vi "Query Current.vi"(8 "error in (no error)":errorcluster, 11 "Manual PSU in":refnum<class "Manual PSU.lvclass">) -> (0 "error out":errorcluster, 2 "Current":dbl, 3 "Manual PSU out":refnum<class "Manual PSU.lvclass">)   [LabVIEW 2020, in "Manual PSU.lvclass"]
uses:
  Manual PSU.lvclass
  C:/Sandbox/Git_Sandbox/WiSpry Test Framework source code (LV20)/WiSpry Test Framework/Instruments/Power Supply/Power Supply.lvclass
  Power Supply.lvclass/Power Supply.ctl
  Power Supply.lvclass
panel:
  out "OK":bool
  in  "Enable":bool=TRUE
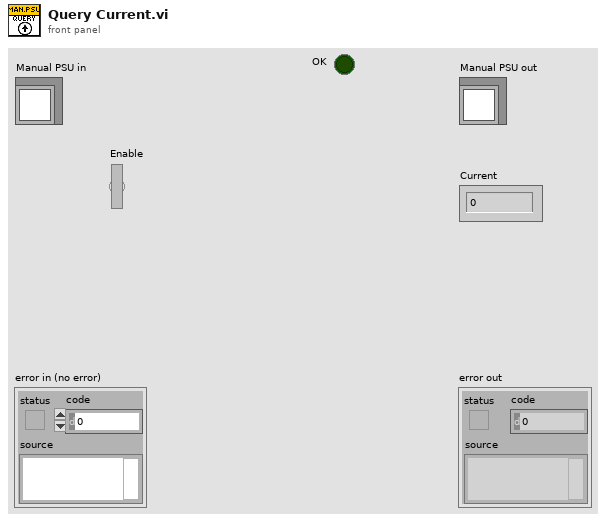
[diagram p1: front panel]
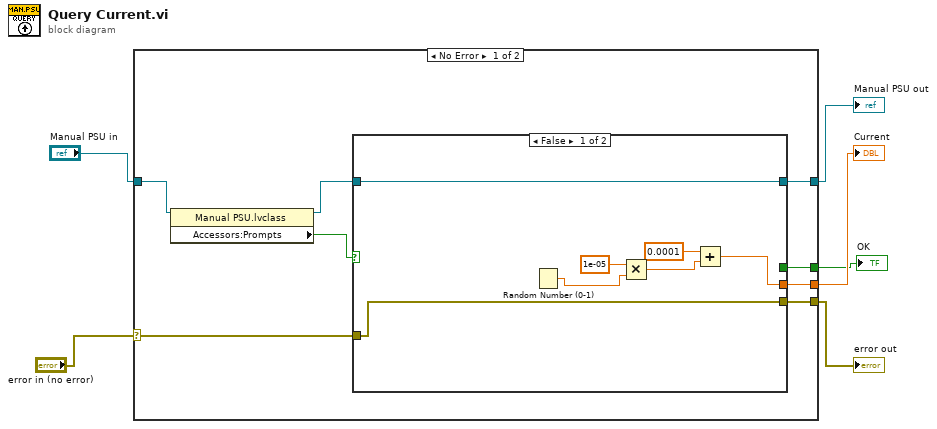
[diagram p0: block diagram]
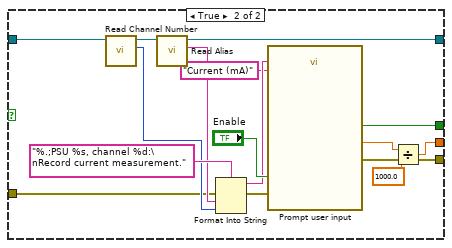
[diagram p2: hidden frame]
diagram:
  n1 = case shown="No Error" "error in (no error)" {
    selector: "error in (no error)" -> [w11 w38]
    tunnel: "Manual PSU in" -> [w9 w39]
    tunnel: [w14 w39] -> w4
    tunnel: [w10 _] -> w2
    tunnel: [w13 w38] -> w3
    tunnel: [w12 _] -> w1
    frame No Error {
      n2 = property class="Manual PSU.lvclass"(reference=w9) -> (reference out=w8:refnum<class "Manual PSU.lvclass">, "Accessors:Prompts"=w7:bool)  [unwired: 1 in, 1 out]
      n3 = case shown="False" w7 {
        tunnel: w8 -> [w20 w36]
        tunnel: [w20 w35] -> w14
        tunnel: [w21 w34] -> w13
        tunnel: [_ w32] -> w12
        tunnel: w11 -> [w21 w26]
        tunnel: [w17 w22] -> w10
        frame False {
          n4 = Random Number (0-1)() -> (number: 0 to 1=w19:dbl)
          n5 = Multiply(x=1e-05, y=w19) -> (x*y=w18:dbl)
          n6 = Add(x=0.0001, y=w18) -> (x+y=w17:dbl)
        }
        frame True {
          n7 = call "Read Channel Number.vi"("Power Supply in"=w36) -> ("Channel Number"=w29:u8, "Power Supply out"=w37:refnum<class "Manual PSU.lvclass">)  [unwired: 9 in]
          n8 = call-dynamic "Read Alias.vi"("Power Supply in"=w37) -> ("Alias"=w30:string, "Power Supply out"=w35:refnum<class "Manual PSU.lvclass">)  [unwired: 9 in]
          n9 = Format Into String(format string="%.;PSU %s, channel %d:\nRecord current measurement.", error in=w26, w30, w29) -> (resulting string=w27:string, error out=w28:errorcluster)  [unwired: 1 in]
          n10 = call "Prompt user input.vi"("Enable"="Enable", "String"=w27, "Parameter Caption"="Current (mA)", "error in (no error)"=w28) -> ("output"=w24:dbl, "OK"=w32:bool, "error out"=w34:errorcluster)  [unwired: 13 in]
          n11 = Divide(x=w24, y=1000.0) -> (x/y=w22:dbl)
        }
      }
    }
    frame Error {
    }
  }
  "error out" <- w3
  "Manual PSU out" <- w4
  "Current" <- w2
  "OK" <- w1
